vi "Register Worker.vi"(8 "error in (no error)":errorcluster, 10 "Worker":refnum<class "Job Handler.lvclass">, 11 "Mock Job Handler In":refnum<class "Mock Job Handler.lvclass">) -> (0 "error out":errorcluster, 3 "Mock Job Handler Out":refnum<class "Mock Job Handler.lvclass">)   [LabVIEW 2020, in "Mock Job Handler.lvclass"]
uses:
  Mock Job Handler.lvclass
  Processes/People/Process Job/Job Handler.lvclass
  Mock Job Handler.lvclass/Mock Job Handler.ctl
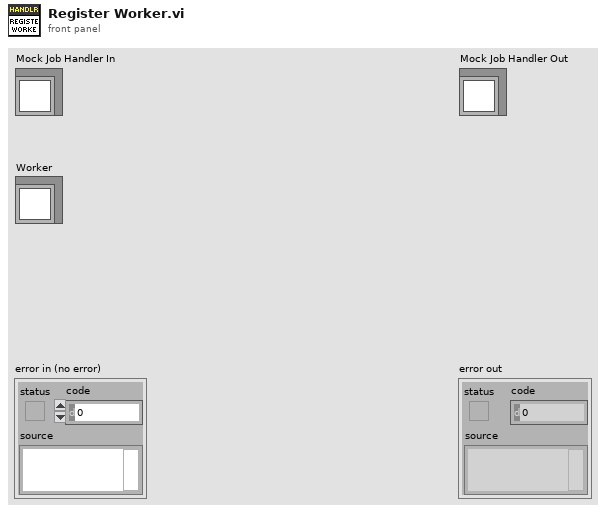
[diagram p1: front panel]
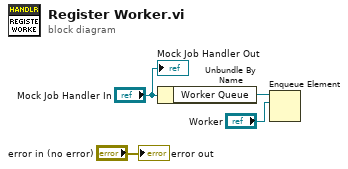
[diagram p0: block diagram]
diagram:
  n1 = Unbundle By Name("Mock Job Handler In") -> ("Worker Queue"=w3:refnum<queue>)
  n2 = Enqueue Element(queue=w3, element="Worker") -> ()  [unwired: 2 in, 3 out]
  "error out" <- "error in (no error)"
  "Mock Job Handler Out" <- "Mock Job Handler In"
